vi "Ventil_bool_to_ring.vi"(8 "ZU":bool, 11 "AUF":bool) -> (3 "ring":i32)   [LabVIEW 2011]
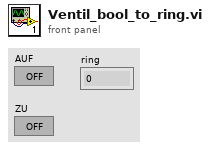
[diagram p1: front panel]
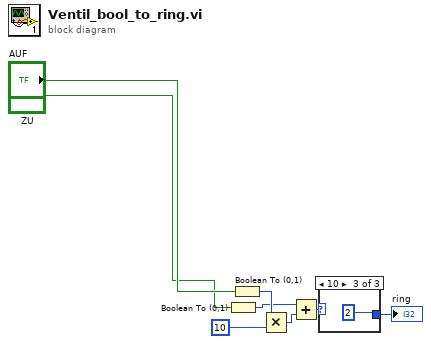
[diagram p0: block diagram]
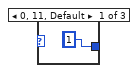
[diagram p2: hidden frame]
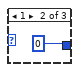
[diagram p3: hidden frame]
diagram:
  n1 = Boolean To (0,1)(Boolean="ZU") -> (0, 1=w2:i16)
  n2 = Boolean To (0,1)(Boolean="AUF") -> (0, 1=w4:i16)
  n3 = Multiply(x=w4, y=i16 10) -> (x*y=w3:i16)
  n4 = Add(x=w2, y=w3) -> (x+y=w6:i16)
  n5 = case shown="10" w6 {
    tunnel: [1 ("V-14 2") 0 ("V-14 2") 2 ("V-14 2")] -> w1
    frame 0, 11, Default {
      (unwired) i16 1 ("y")
    }
    frame 1 {
    }
    frame 10 {
    }
  }
  "ring" <- w1
